vi "to_byte_string.vi"(11 "Bytes in":refnum<class "Bytes.lvclass">) -> (3 "byte string":string)   [LabVIEW 2020, in "variant.lvlib" / "Bytes.lvclass"]
uses:
  Bytes.lvclass
  Bytes.lvclass/Bytes.ctl
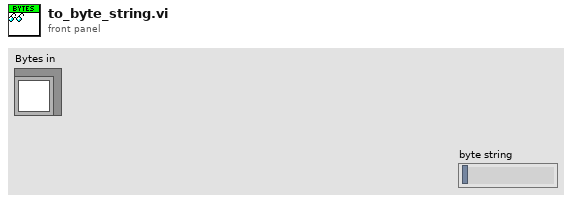
[diagram p1: front panel]
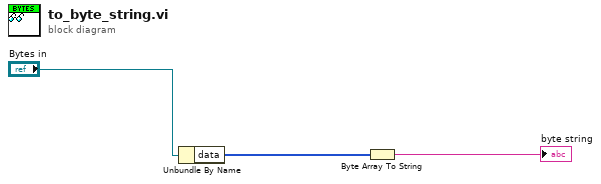
[diagram p0: block diagram]
diagram:
  n1 = Unbundle By Name("Bytes in") -> ("data"=w2:u8[])
  n2 = Byte Array To String(unsigned byte array=w2) -> (string=→"byte string":string)
